vi "Cluster_ref_generator.vi"(0 "Cluster":T1={"IP Address"=["", "", "", "", "", "", "", "", "", ""], "Machine name"=["", "", "", "", "", "", "", "", "", ""], "Station number"=["", "", "", "", "", "", "", "", "", ""], "Product List"=[], "Recipe_upload_history path"=path "", "reference"=refnum, "appended array"=[]}, 1 "CtlRef":refnum<vi>, 2 "Index from Cluster":i32=1, 3 "error in (no error)":errorcluster, 6 "Type":enum16{"String", "Numeric", "Boolean", ""}(ring)=enum."Boolean") -> (7 "Value":variant, 10 "error out":errorcluster)   [LabVIEW 2017]
uses:
  Controls/cluster.ctl
  <vilib>/addons/database/Connection.llb/Conn ObjectReference.ctl
  <vilib>/addons/database/NI_Database_API.lvlib
panel:
  in  "Numeric":i64
  in  "Boolean":bool
  in  "String":string
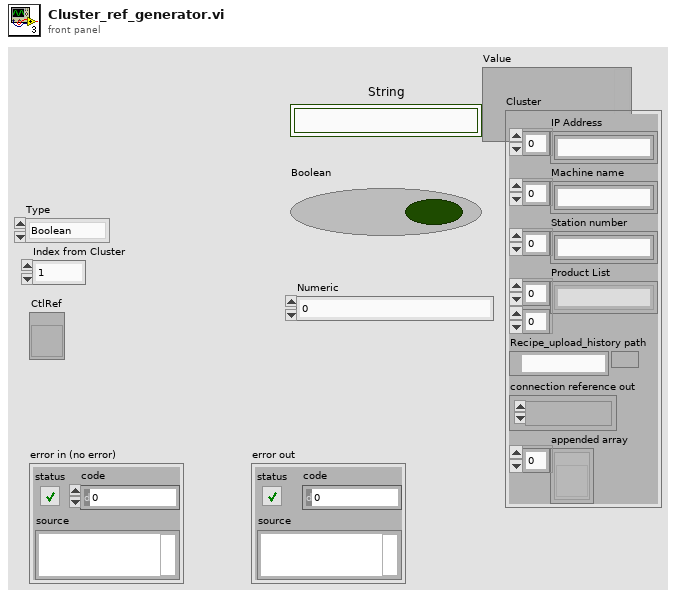
[diagram p1: front panel]
types:
  T1 = typedef "cluster.ctl" = cluster{"IP Address":string[], "Machine name":string[], "Station number":string[], "Product List":string[][], "Recipe_upload_history path":path, "reference":T2, "appended array":refnum<vi>[]}
  T2 = typedef "NI_Database_API.lvlib/Conn ObjectReference.ctl" = refnum<k1>
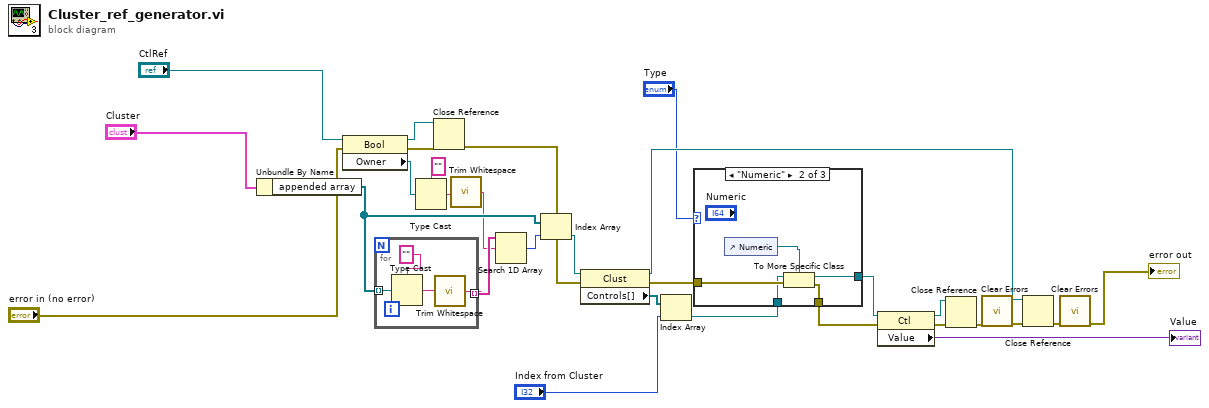
[diagram p0: block diagram]
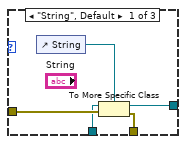
[diagram p2: hidden frame]
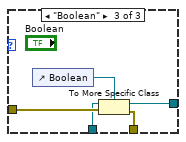
[diagram p3: hidden frame]
diagram:
  n1 = Unbundle By Name("Cluster") -> ("appended array"=w24:refnum<vi>[])
  n2 = property class="Bool"(reference="CtlRef", error in="error in (no error)") -> (reference out=w6:refnum<vi>, error out=w7:errorcluster, "Owner"=w11:refnum<vi>)
  n3 = for {
    tunnel: w24 -> [w33] mode=indexing
    tunnel: [w30] -> w13 mode=indexing
    n4 = Type Cast(type="" ("String"), x=w33) -> (*(type *) &x=w31:string)
    n5 = call <vilib>:"Trim Whitespace.vi"("string"=w31) -> ("trimmed string"=w30:string)  [unwired: 1 in]
  }
  n6 = Type Cast(type="", x=w11) -> (*(type *) &x=w10:string)
  n7 = Close Reference(reference=w6, error in (no error)=w7) -> (error out=w26:errorcluster)
  n8 = call <vilib>:"Trim Whitespace.vi"("string"=w10) -> ("trimmed string"=w12:string)  [unwired: 1 in]
  n9 = Search 1D Array(1D array=w13, element=w12) -> (index of element=w23:i32)  [unwired: 1 in]
  n10 = Index Array(array=w24, index=w23) -> (element=w25:refnum<vi>)
  n11 = property on="Property Node" class="Clust"(reference=w25, error in=w26) -> (reference out=w20:refnum<vi>, error out=w27:errorcluster, "Controls[]"=w14:refnum<vi>[])
  n12 = Index Array(array=w14, index="Index from Cluster") -> (element=w16:refnum<vi>)
  n13 = case shown="\"Numeric\"" "Type" {
    tunnel: [w38 w43 w48] -> w28
    tunnel: w27 -> [w37 w42 w47]
    tunnel: [w36 w41 w46] -> w17
    tunnel: w16 -> [w35 w40 w45]
    frame "String", Default {
      n14 = control-ref of="String"() -> (w34:refnum<vi>)
      n15 = To More Specific Class(target class=w34, reference=w35, error in=w37) -> (specific class reference=w36:refnum<vi>, error out=w38:errorcluster)
    }
    frame "Numeric" {
      n16 = control-ref of="Numeric"() -> (w39:refnum<vi>)
      n17 = To More Specific Class(target class=w39, reference=w40, error in=w42) -> (specific class reference=w41:refnum<vi>, error out=w43:errorcluster)
    }
    frame "Boolean" {
      n18 = control-ref of="Boolean"() -> (w44:refnum<vi>)
      n19 = To More Specific Class(target class=w44, reference=w45, error in=w47) -> (specific class reference=w46:refnum<vi>, error out=w48:errorcluster)
    }
  }
  n20 = property on="Property Node" class="Ctl"(reference=w17, error in=w28) -> (reference out=w18:refnum<vi>, error out=w19:errorcluster, "Value"=→"Value":variant)
  n21 = Close Reference(reference=w18, error in (no error)=w19) -> (error out=w21:errorcluster)
  n22 = call <vilib>:"Clear Errors.vi"("error in (no error)"=w21) -> ("error out"=w22:errorcluster)  [unwired: 5 in, 1 out]
  n23 = Close Reference(reference=w20, error in (no error)=w22) -> (error out=w29:errorcluster)
  n24 = call <vilib>:"Clear Errors.vi"("error in (no error)"=w29) -> ("error out"=→"error out":errorcluster)  [unwired: 5 in, 1 out]
